vi "Cache.TestSteps.Read.vi"(7 "Idx":i32, 8 "error in (no error)":errorcluster, 10 "Ref":string) -> (0 "error out":errorcluster, 2 "TS in":T1 {"TS"."TP"."value" format="%#.3f"; "TS"."TV"."minimum" format="%#.3f"; "TS"."TV"."maximum" format="%#.3f"})   [LabVIEW 2016]
uses:
  Cache.TestSteps.Fglb.TestData.ctl
  Database/ProdaNG/Controls/ProdaNG.Process.ctl
  Database/ProdaNG/Controls/ProdaNG.ProcessStep.ctl
  Database/ProdaNG/Controls/ProdaNG.ProcessStepParam.ctl
  Database/ProdaNG/Controls/ProdaNG.TestStep.ctl
  Database/ProdaNG/Controls/ProdaNG.TestValue.ctl
  Database/ProdaNG/Controls/ProdaNG.TestStepParam.ctl
  Database/ProdaNG/Controls/ProdaNG.Unit.ctl
  Global/ApplicationGlobal.vi
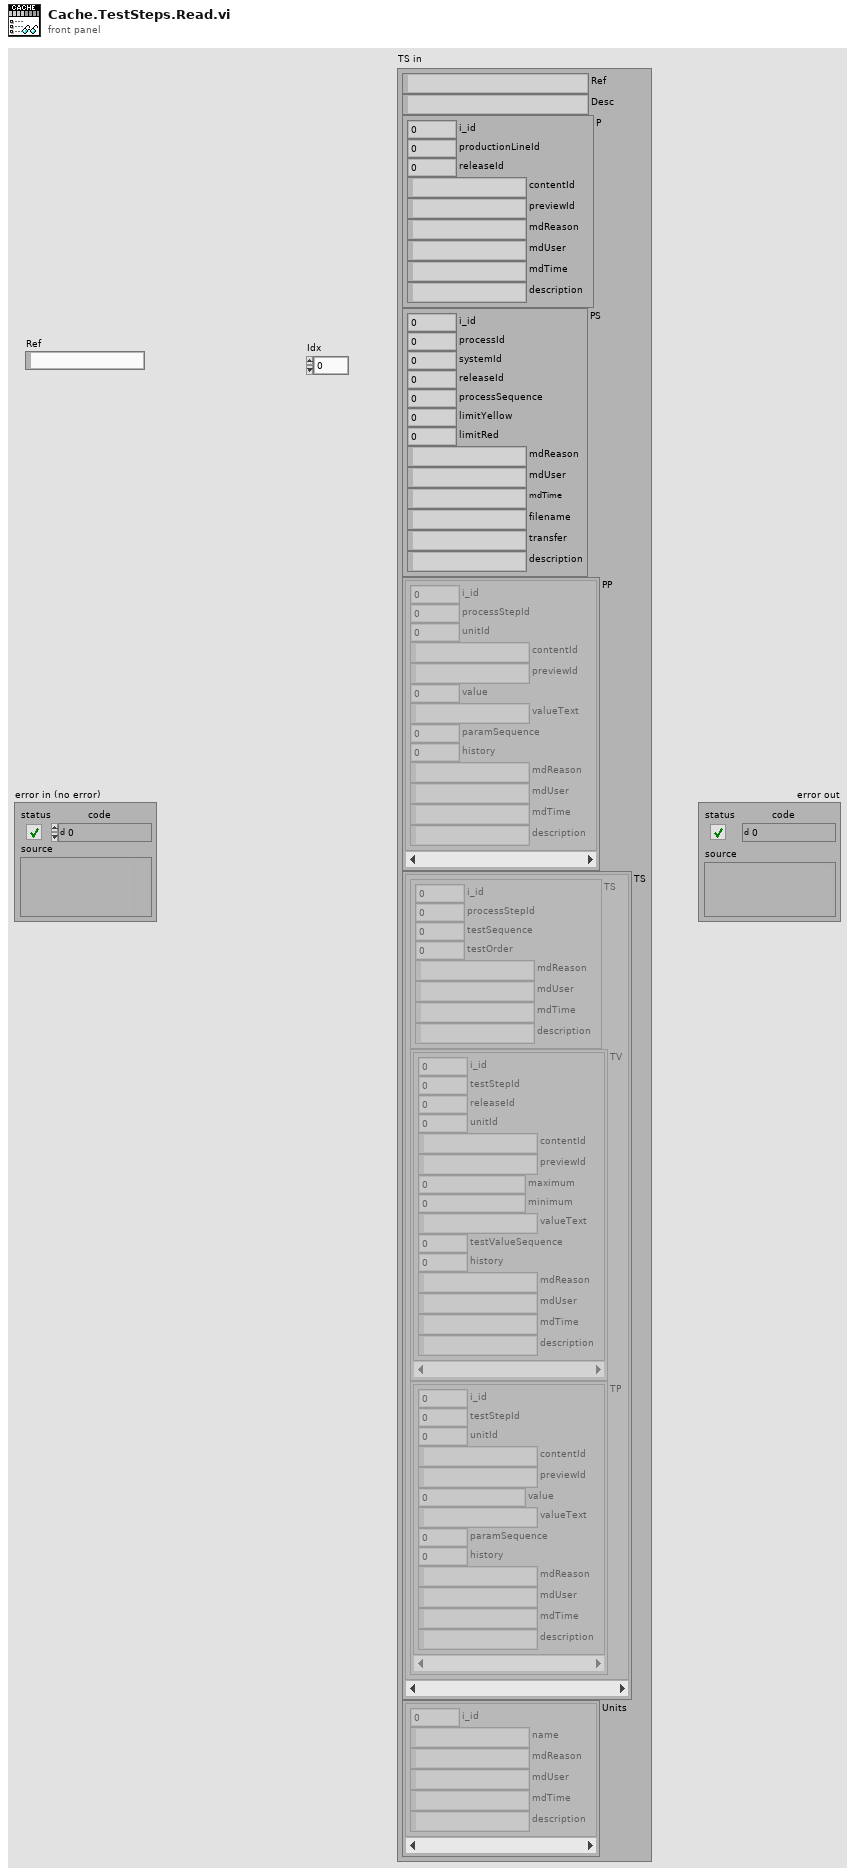
[diagram p1: front panel]
types:
  T1 = typedef "Cache.TestSteps.Fglb.TestData.ctl" = cluster{"Ref":string, "Desc":string, "P":T2, "PS":T3, "PP":T4[], "TS":cluster{"TS":T5, "TV":T6[], "TP":T7[]}[], "Units":T8[]}
  T2 = typedef "ProdaNG.Process.ctl" = cluster{"i_id":i32, "productionLineId":i32, "releaseId":i32, "contentId":string, "previewId":string, "mdReason":string, "mdUser":string, "mdTime":string, "description":string}
  T3 = typedef "ProdaNG.ProcessStep.ctl" = cluster{"i_id":i32, "processId":i32, "systemId":i32, "releaseId":i32, "processSequence":i32, "limitYellow":dbl, "limitRed":dbl, "mdReason":string, "mdUser":string, "mdTime":string, "filename":string, "transfer":string, "description":string}
  T4 = typedef "ProdaNG.ProcessStepParam.ctl" = cluster{"i_id":i32, "processStepId":i32, "unitId":i32, "contentId":string, "previewId":string, "value":dbl, "valueText":string, "paramSequence":i32, "history":i32, "mdReason":string, "mdUser":string, "mdTime":string, "description":string}
  T5 = typedef "ProdaNG.TestStep.ctl" = cluster{"i_id":i32, "processStepId":i32, "testSequence":i32, "testOrder":i32, "mdReason":string, "mdUser":string, "mdTime":string, "description":string}
  T6 = typedef "ProdaNG.TestValue.ctl" = cluster{"i_id":i32, "testStepId":i32, "releaseId":i32, "unitId":i32, "contentId":string, "previewId":string, "maximum":dbl, "minimum":dbl, "valueText":string, "testValueSequence":i32, "history":i32, "mdReason":string, "mdUser":string, "mdTime":string, "description":string}
  T7 = typedef "ProdaNG.TestStepParam.ctl" = cluster{"i_id":i32, "testStepId":i32, "unitId":i32, "contentId":string, "previewId":string, "value":dbl, "valueText":string, "paramSequence":i32, "history":i32, "mdReason":string, "mdUser":string, "mdTime":string, "description":string}
  T8 = typedef "ProdaNG.Unit.ctl" = cluster{"i_id":i32, "name":string, "mdReason":string, "mdUser":string, "mdTime":string, "description":string}
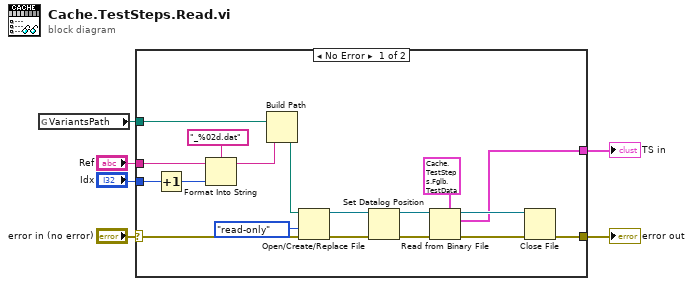
[diagram p0: block diagram]
diagram:
  n1 = global read "ApplicationGlobal.vi" "VariantsPath"() -> (w4:path)
  n2 = case shown="No Error" "error in (no error)" {
    selector: "error in (no error)" -> [w22 w25]
    tunnel: [w18 w25] -> w5
    tunnel: [w15 _] -> w1
    tunnel: w4 -> [w13 _]
    tunnel: "Idx" -> [w12 _]
    tunnel: "Ref" -> [w11 _]
    frame No Error {
      n3 = Increment(x=w12) -> (x+1=w7:i32)
      n4 = Format Into String(format string="_%02d.dat", initial string=w11, w7) -> (resulting string=w9:string)  [unwired: 1 in, 1 out]
      n5 = Build Path(base path=w13, name or relative path=w9) -> (appended path=w10:path)
      n6 = Open/Create/Replace File(file path (use dialog)=w10, error in=w22, access (0:read/write)=enum16{"read/write", "read-only", "write-only"}."read-only") -> (refnum out=w17:refnum<file>, error out=w16:errorcluster)  [unwired: 3 in, 1 out]
      n7 = Set Datalog Position(4:w16, 7:w17) -> (0:w24:errorcluster, 3:w23:refnum<file>)  [unwired: 2 in]
      n8 = Read from Binary File(5:T1 {"Ref"="", "Desc"="", "P"={"i_id"=0, "productionLineId"=0, "releaseId"=0, "contentId"="", "previewId"="", "mdReason"="", "mdUser"="", "mdTime"="", "description"=""}, "PS"={"i_id"=0, "processId"=0, "systemId"=0, "releaseId"=0, "processSequence"=0, "limitYellow"=0.0, "limitRed"=0.0, "mdReason"="", "mdUser"="", "mdTime"="", "filename"="", "transfer"="", "description"=""}, "PP"=[], "TS"=[], "Units"=[]} ("TS in"), 8:w24, 11:w23) -> (0:w19:errorcluster, 2:w15:T1, 3:w20:refnum<file>)  [unwired: 3 in, 1 out]
      n9 = Close File(refnum=w20, error in=w19) -> (error out=w18:errorcluster)  [unwired: 1 out]
    }
    frame Error {
    }
  }
  "error out" <- w5
  "TS in" <- w1
